vi "Fridge Variable.vi"() -> ()   [LabVIEW 2010]
panel:
  out "Fridge Array":dbl[](array[numeric])
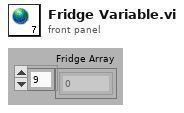
[diagram p1: front panel]
diagram:
